vi "L1_RegisterDa_File_Appender.vi"(0 "Vin":dbl, 1 "file path (dialog if empty)":path, 5 "CH":dbl, 7 "Active Adder":dbl, 9 "DAC Level":dbl=63.0, 11 "Vmeas":dbl, 12 "IPR":dbl) -> ()   [LabVIEW 2012]
uses:
  <vilib>/Utility/file.llb/Write To Spreadsheet File (string).vi
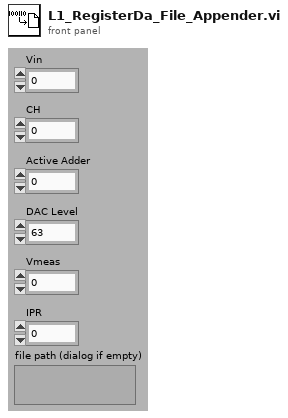
[diagram p1: front panel]
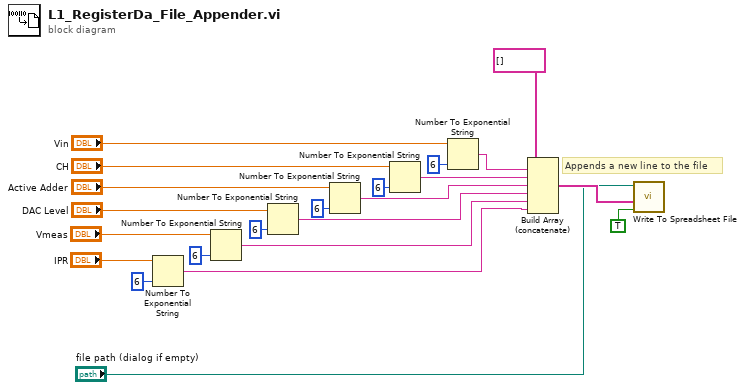
[diagram p0: block diagram]
diagram:
  # "Appends a new line to the file"
  n1 = Number To Exponential String(number="IPR", precision (6)=i16 6) -> (E-format string=w1:string)  [unwired: 2 in]
  n2 = Number To Exponential String(number="Vmeas", precision (6)=i16 6) -> (E-format string=w4:string)  [unwired: 2 in]
  n3 = Number To Exponential String(number="DAC Level", precision (6)=i16 6) -> (E-format string=w19:string)  [unwired: 2 in]
  n4 = Number To Exponential String(number="Active Adder", precision (6)=i16 6) -> (E-format string=w21:string)  [unwired: 2 in]
  n5 = Number To Exponential String(number="CH", precision (6)=i16 6) -> (E-format string=w22:string)  [unwired: 2 in]
  n6 = Number To Exponential String(number="Vin", precision (6)=i16 6) -> (E-format string=w15:string)  [unwired: 2 in]
  n7 = Build Array (concatenate)(string[] [] ("array"), w15, w22, w21, w19, w4, w1) -> (w11:string[])
  n8 = call-poly <vilib>:"Write To Spreadsheet File.vi"("append to file? (new file:F)"=TRUE, "1D data"=w11, "file path (dialog if empty)"="file path (dialog if empty)") -> ()  [unwired: 5 in, 1 out]
